vi "Split RegisterMap into Controls and Indicators.vi"(10 "RegisterMap":T2[](array[typedef]) {"Address" format="%.0x"}) -> (1 "Controls":T1[](array[typedef]) {"reservation info"."reserver ref in" format="%.0x"; "Register Info"."Address" format="%.0x"}, 3 "Indicators":T1[](array[typedef]) {"reservation info"."reserver ref in" format="%.0x"; "Register Info"."Address" format="%.0x"})   [LabVIEW 2016, in "FPGA Addon System Explorer.lvlib"]
uses:
  FPGA Addon System Explorer.lvlib
  <vilib>/rvi/Bitfile/nirviControlStructure.ctl
  <vilib>/rvi/Bitfile/nirviTypdefDescription.ctl
  <vilib>/rvi/Bitfile/nirviMechanicalAction.ctl
  <vilib>/rvi/Bitfile/nirviSubControlStructure.ctl
  <vilib>/rvi/Bitfile/nirviClusterElementControl.ctl
  SubVIs/Register Reservation.ctl
  SubVIs/reservation info.ctl
  <vilib>/NI Veristand/Custom Device API/Custom Device Item Ref.ctl
  <vilib>/NI VeriStand/Custom Device API/Custom Device API.lvlib
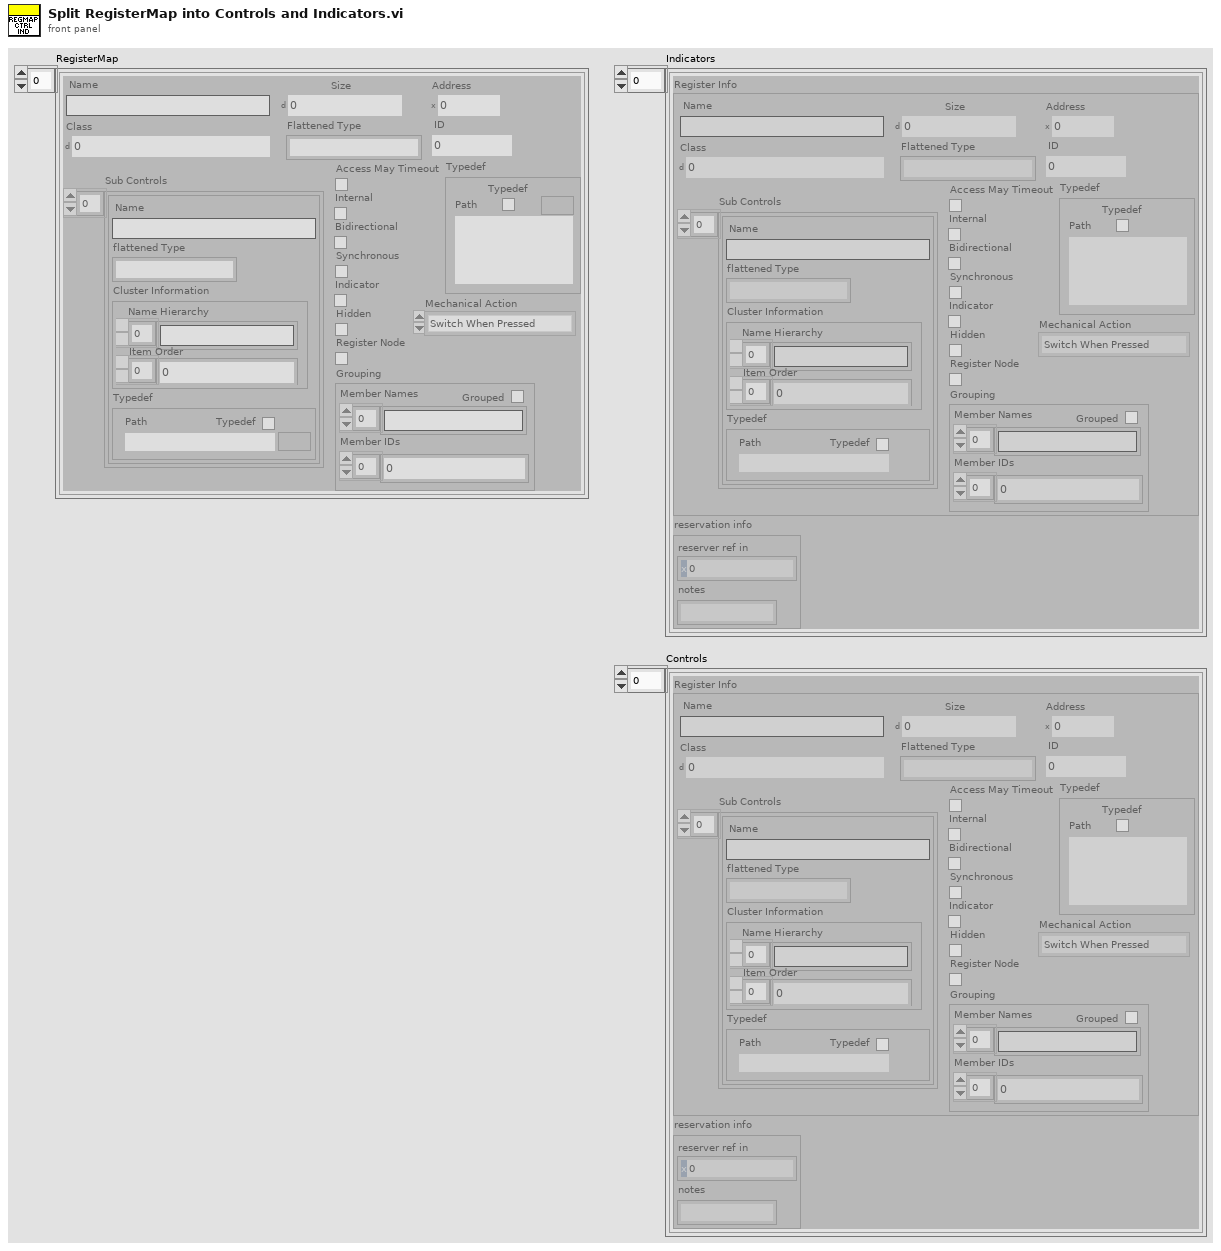
[diagram p1: front panel]
types:
  T1 = typedef "FPGA Addon System Explorer.lvlib/Register Reservation.ctl" = cluster{"Register Info":T2, "reservation info":T7}
  T2 = typedef "nirviControlStructure.ctl" = cluster{"Name":string, "Hidden":bool, "Indicator":bool, "Flattened Type":string, "Grouping":cluster{"Grouped":bool, "Member Names":string[], "Member IDs":u32[]}, "Address":u32, "Size":u32, "Class":u32, "Internal":bool, "Typedef":T3, "ID":u32, "Bidirectional":bool, "Synchronous":bool, "Mechanical Action":T4, "Sub Controls":T5[], "Access May Timeout":bool, "Register Node":bool}
  T3 = typedef "nirviTypdefDescription.ctl" = cluster{"Typedef":bool, "Path":path}
  T4 = typedef "nirviMechanicalAction.ctl" = enum8{"Switch When Pressed", "Switch When Released", "Switch Until Released", "Latch When Pressed", "Latch When Released", "Latch Until Released"}
  T5 = typedef "nirviSubControlStructure.ctl" = cluster{"Name":string, "flattened Type":string, "Cluster Information":T6, "Typedef":T3}
  T6 = typedef "nirviClusterElementControl.ctl" = cluster{"Name Hierarchy":string[], "Item Order":u32[]}
  T7 = typedef "FPGA Addon System Explorer.lvlib/reservation info.ctl" = cluster{"reserver ref in":T8, "notes":string}
  T8 = typedef "Custom Device API.lvlib/Custom Device Item Ref.ctl" = u64
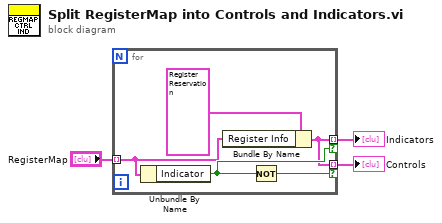
[diagram p0: block diagram]
diagram:
  n1 = for {
    tunnel: "RegisterMap" -> [w5] mode=indexing
    tunnel: [w4] -> w1 mode=indexing if=w8
    tunnel: [w4] -> w2 mode=indexing if=w7
    n2 = Unbundle By Name(w5) -> ("Indicator"=w7:bool)
    n3 = Bundle By Name(cluster=T1 {"Register Info"={"Name"="", "Hidden"=FALSE, "Indicator"=FALSE, "Flattened Type"="", "Grouping"={"Grouped"=FALSE, "Member Names"=[], "Member IDs"=[]}, "Address"=0, "Size"=0, "Class"=0, "Internal"=FALSE, "Typedef"={"Typedef"=FALSE, "Path"=path ""}, "ID"=0, "Bidirectional"=FALSE, "Synchronous"=FALSE, "Mechanical Action"=enum."Switch When Pressed", "Sub Controls"=[], "Access May Timeout"=FALSE, "Register Node"=FALSE}, "reservation info"={"reserver ref in"=0, "notes"=""}} ("Cluster"), "Register Info"=w5) -> (w4:T1)
    n4 = Not(x=w7) -> (.not. x?=w8:bool)
  }
  "Indicators" <- w2
  "Controls" <- w1
